vi "Stop Process.vi"(8 "error in (no error)":errorcluster, 11 "Process Model in":refnum<class "Process Model.lvclass">) -> (0 "error out":errorcluster, 3 "Process Model out":refnum<class "Process Model.lvclass">)   [LabVIEW 2017, in "Car Wash.lvlib" / "Process Model.lvlib" / "Process Model.lvclass"]
uses:
  Process Model.lvclass
  <vilib>/ActorFramework/Actor/Actor.lvclass
  <vilib>/ActorFramework/Stop Msg/Stop Msg.lvclass
  D:/Project/General VIs/Process/iProcess Model/iProcess Model/iProcess Model.lvclass
  C:/Program Files/National Instruments/LabVIEW 2017/vi.lib/gpm_packages/@cs/mva-core/Source/IModel/IModel/IModel.lvclass
  C:/Program Files/National Instruments/LabVIEW 2017/vi.lib/gpm_packages/@cs/mva-core/Source/IObserver/IObserver/IObserver.lvclass
  C:/Program Files/National Instruments/LabVIEW 2017/vi.lib/ActorFramework/Actor/Actor.lvclass
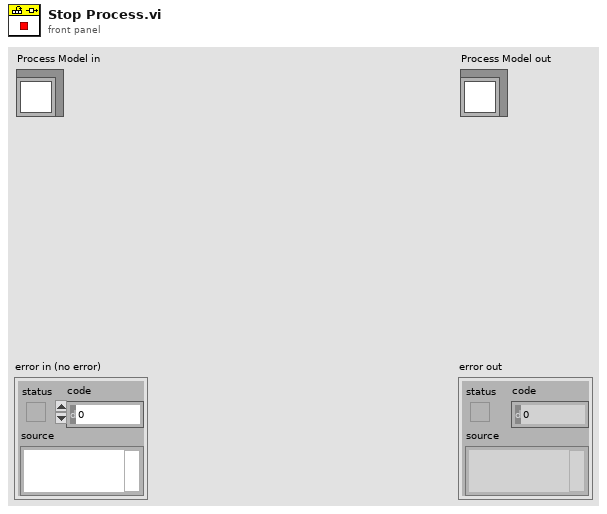
[diagram p1: front panel]
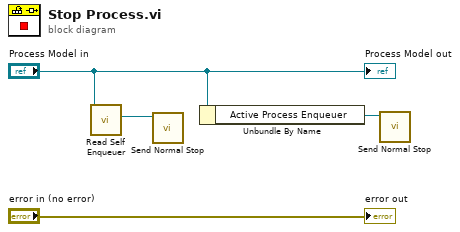
[diagram p0: block diagram]
diagram:
  n1 = call <vilib>:"Read Self Enqueuer.vi"("Actor"="Process Model in") -> ("Self Enqueuer"=w3:refnum<class "Message Enqueuer.lvclass">)  [unwired: 10 in]
  n2 = call <vilib>:"Send Normal Stop.vi"("Message Enqueuer"=w3) -> ()  [unwired: 10 in, 1 out]
  n3 = Unbundle By Name("Process Model in") -> ("Active Process Enqueuer"=w1:refnum<class "Message Enqueuer.lvclass">)
  n4 = call <vilib>:"Send Normal Stop.vi"("Message Enqueuer"=w1) -> ()  [unwired: 10 in, 1 out]
  "error out" <- "error in (no error)"
  "Process Model out" <- "Process Model in"
